vi "Load Help File.vi"(8 "error in (no error)":errorcluster, 9 "HTML File":string="MainPage_J1939.html", 10 "Main CHM File":string="J1939.chm", 11 "SHDocVw.IWebBrowser2":refnum<k7>(container)) -> (0 "error out":errorcluster)   [LabVIEW 2015, in "Modbus Master System Explorer.lvlib"]
uses:
  Modbus Master System Explorer.lvlib
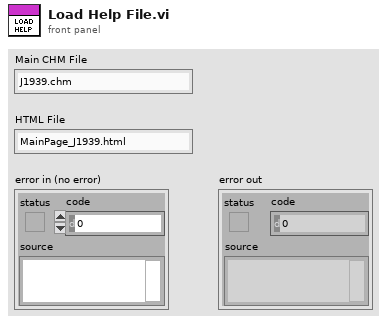
[diagram p1: front panel]
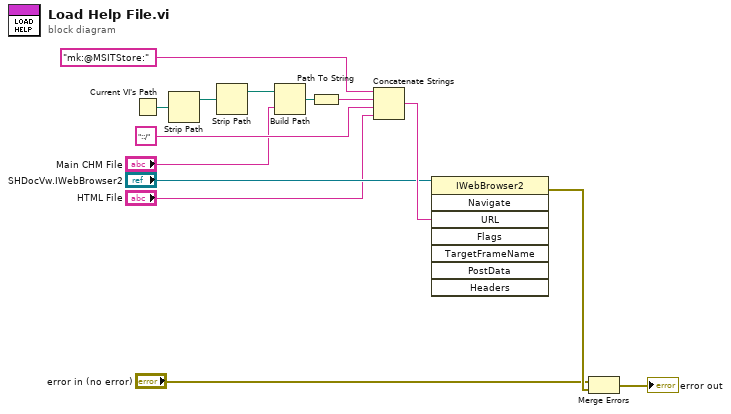
[diagram p0: block diagram]
diagram:
  n1 = Current VI's Path() -> (path=w13:path)
  n2 = Strip Path(path=w13) -> (stripped path=w12:path)  [unwired: 1 out]
  n3 = Strip Path(path=w12) -> (stripped path=w7:path)  [unwired: 1 out]
  n4 = Build Path(base path=w7, name or relative path="Main CHM File") -> (appended path=w9:path)
  n5 = Path To String(path=w9) -> (string=w10:string)
  n6 = Concatenate Strings("mk:@MSITStore:" ("string"), w10, "::/" ("name or relative path"), "HTML File") -> (w6:string)
  n7 = invoke class="IWebBrowser2" method="Navigate"(reference="SHDocVw.IWebBrowser2", "URL"=w6) -> (error out=w3:errorcluster)  [unwired: 6 in, 7 out]
  n8 = Merge Errors("error in (no error)", w3) -> (→"error out":errorcluster)
